vi "Main.vi"(8 "error in":errorcluster, 9 "Error Queue":refnum<queue>, 10 "Controller Queue":refnum<queue>, 11 "Application Events":refnum<user-event>) -> (0 "error out":errorcluster)   [LabVIEW 2020, in "User Console.lvlib"]
uses:
  User Console.lvlib
  Controller/Controls/Module Message.ctl
  Controller/Controls/Application Modules.ctl
  Controller/Controls/Application Event Message.ctl
  Controller/Controls/Application Events.ctl
  Controls/Module Loop Data.ctl
  Controller/Controller.lvlib
panel:
  in  "Door Buttons":cluster{"Door Open":bool, "Door Close":bool}
  in  "Floor Selection":T1
  in  "Elevator Call":T2
  in  "Emergency":bool
  # "[Covers: UI1]"
  # "[Covers: UI2]\n[Covers: UI2A] \n[Covers: UI2A1] \n[Covers: UI2A2] \n[Covers: UI2B] \n[Covers: UI2B1] \n[Covers: UI2B2] \n[Covers: UI2C] \n[Covers: UI2C1] \n[Covers: UI2C2] \n[Covers: UI2C3]"
  # "[Covers: UI2D] \n[Covers: UI2D1]"
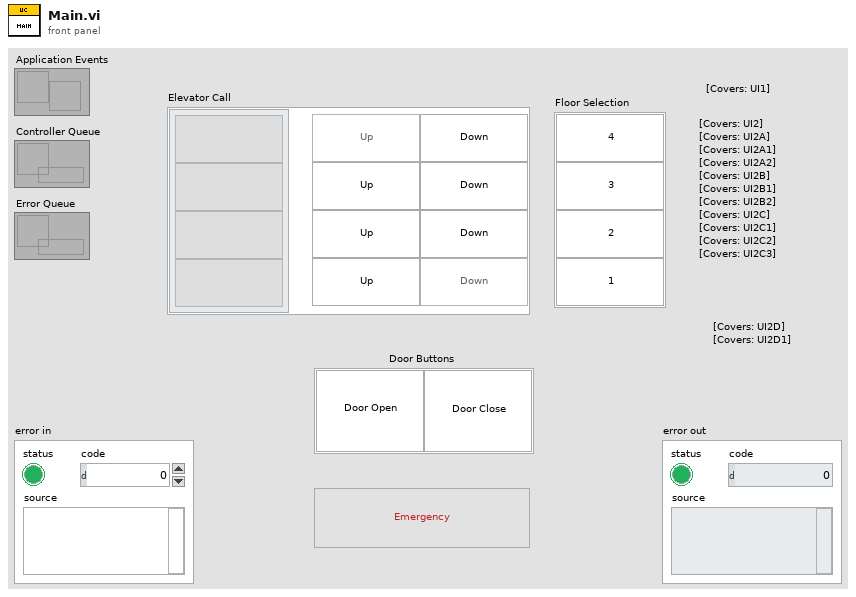
[diagram p1: front panel]
types:
  T1 = cluster{"Floor 1":bool, "Floor 2":bool, "Floor 3":bool, "Floor 4":bool}
  T2 = cluster{"Up Floor 1 ":bool, "Up Floor 2":bool, "Up Floor 3":bool, "Up Floor 4":bool, "Down Floor 1":bool, "Down Floor 2":bool, "Down Floor 3":bool, "Down Floor 4":bool, "Floors":string[]}
  T3 = typedef "Controller.lvlib/Application Events.ctl" = enum16{"Controller: Initialize", "Controller: Initialize Start And Move State", "Controller: Initialize Analysis State", "Controller: Initialize Continue Travel State", "Controller: Initialize Stop At Floor", "Controller: Initialize Open And Close Door Sequence", "Controller: Initialize No Request Remaining", "Controller: Initialize Emergency Call", "Controller: Initialize Terminate Process", "Controller: Publish State", "UI: Elevator Call", "UI: Broadcast State", "UI: Next Destination Reached", "UI: Timeout Reached", "UI: Emergency Call", "UI: Terminate State", "UI: Door Opened", "UI: Door Closed", "UI: Floor Reached", "UI: Door About To Close"}
  T4 = typedef "User Console.lvlib/Module Loop Data.ctl" = cluster{"Timing":cluster{"IsTiming?":bool, "Time Target Sec":dbl, "Time Ticks Ms":i32, "Time Ticks Counter":i32}}
  T5 = typedef "Controller.lvlib/Application Event Message.ctl" = cluster{"Source":T6, "Event":T3, "Data":variant}
  T6 = typedef "Controller.lvlib/Application Modules.ctl" = enum16{"Controller", "User Console", "Display Console", "Sensor Interface", "Configuration Database", "Error Module"}
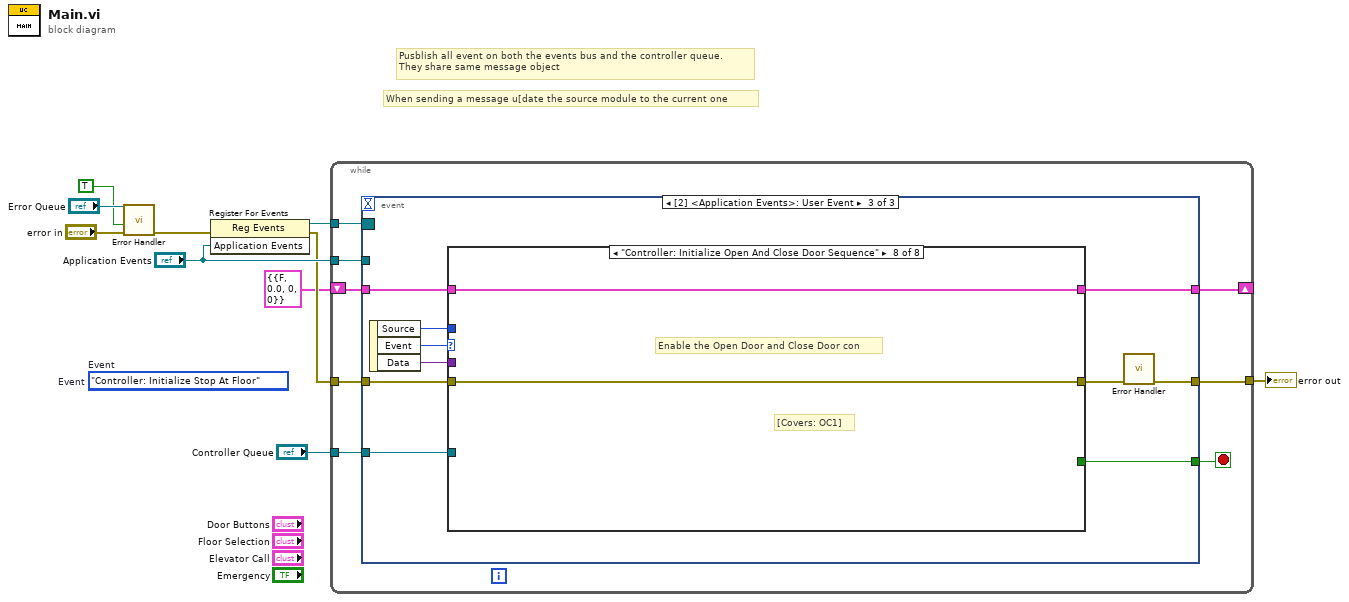
[diagram p0: block diagram]
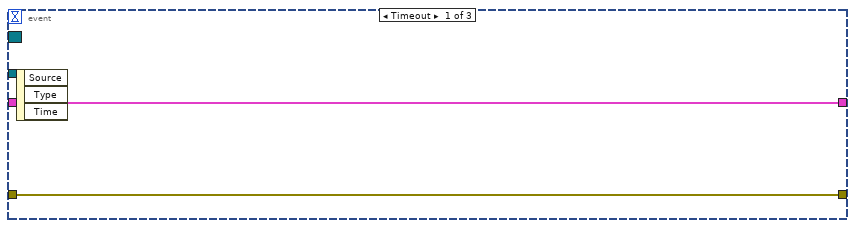
[diagram p2: hidden frame]
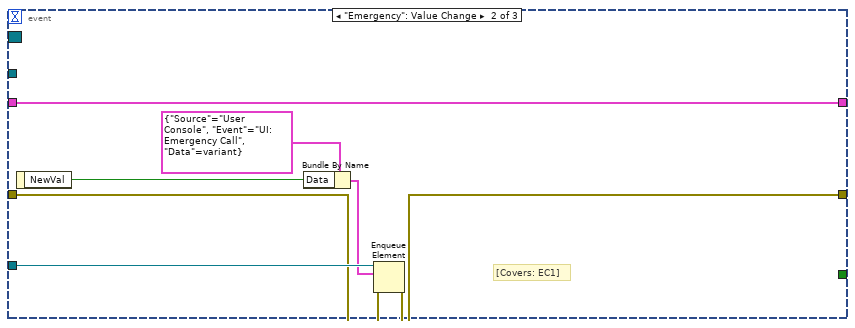
[diagram p3: hidden frame]
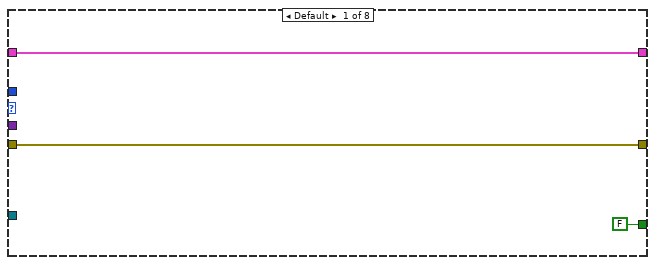
[diagram p4: hidden frame]
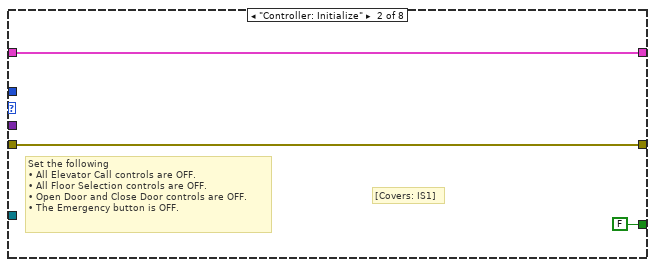
[diagram p5: hidden frame]
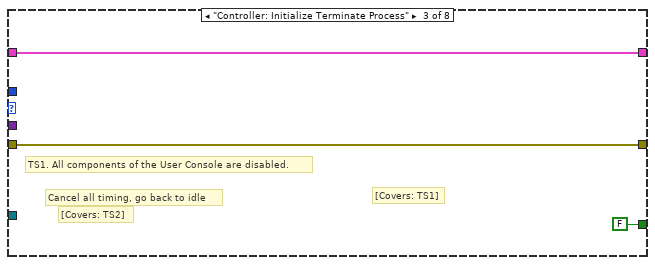
[diagram p6: hidden frame]
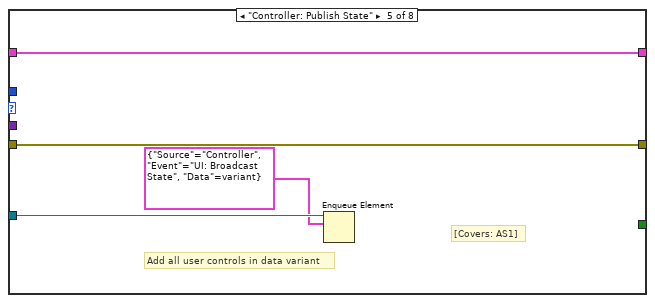
[diagram p8: hidden frame]
diagram:
  (unwired) Application_Events."Controller: Initialize Stop At Floor"  # Event
  (unwired) Application_Events."Controller: Initialize Stop At Floor"  # Event
  # "Pusblish all event on both the events bus and the controller queue. \nThey share same message object"
  # "When sending a message u[date the source module to the current one"
  n1 = call "Error Handler.vi"("error in"="error in", "Load Reference?"=TRUE, "Error Queue"="Error Queue") -> ("error out"=w4:errorcluster)  [unwired: 8 in]
  n2 = register-events(error in=w4, "Application Events") -> (reference out=w9:refnum<event-registration>, error out=w3:errorcluster)  [unwired: 1 in]
  n3 = while {
    tunnel: "Application Events" -> [w18]
    tunnel: w9 -> [w17]
    tunnel: w3 -> [w16]
    tunnel: "Controller Queue" -> [w15]
    tunnel: [w13] -> w2
    shift-right: [w11] -> _
    shift-left: T4 {"Timing"={"IsTiming?"=FALSE, "Time Target Sec"=0.0, "Time Ticks Ms"=0, "Time Ticks Counter"=0}} -> [w12]
    stop <- w14 stop-if-true
    n4 = event shown="[2] <Application Events>: User Event" {
      selector: w17 -> [_ _ _]
      dyn-events: _ -> [_ _ _]
      timeout: _ -> [_ _ _]
      tunnel: w18 -> [_ _ _]
      tunnel: w16 -> [w20 w26 w33]
      tunnel: w15 -> [_ w27 w28]
      tunnel: [_ _ w34] -> w14
      tunnel: [w20 w25 w31] -> w13
      tunnel: w12 -> [w19 w21 w30]
      tunnel: [w19 w21 w29] -> w11
      event Timeout {
        n5 = event-data() -> ()  [unwired: 1 in, 3 out]
      }
      event "Emergency": Value Change {
        # "[Covers: EC1]"
        n6 = event-data() -> ("NewVal"=w24:bool)  [unwired: 1 in]
        n7 = Bundle By Name(cluster=T5 {"Source"=enum."User Console", "Event"=enum."UI: Emergency Call", "Data"=variant} ("element"), "Data"=w24) -> (w22:T5)
        n8 = Enqueue Element(queue=w27, element=w22, error in (no error)=w26) -> (error out=w25:errorcluster)  [unwired: 1 in, 2 out]
      }
      event User Event {
        n9 = event-data() -> ("Source"=w36:T6, "Event"=w37:T3, "Data"=w35:variant)  [unwired: 1 in]
        n10 = case shown="\"Controller: Initialize Open And Close Door Sequence\"" w37 {
          tunnel: w36 -> [_ _ _ _ _ _ _ _]
          tunnel: w35 -> [_ _ _ _ _ _ _ _]
          tunnel: [FALSE FALSE FALSE _ _ _ _ _] -> w34
          tunnel: [w39 w42 w45 w48 w52 w54 w56 w58] -> w32
          tunnel: w33 -> [w39 w42 w45 w48 w52 w54 w56 w58]
          tunnel: w30 -> [w38 w41 w44 w47 w51 w53 w55 w57]
          tunnel: [w38 w41 w44 w47 w51 w53 w55 w57] -> w29
          tunnel: w28 -> [_ _ _ _ w50 _ _ _]
          frame Default {
          }
          frame "Controller: Initialize" {
            # "[Covers: IS1]"
            # "Set the following\n• All Elevator Call controls are OFF.\n• All Floor Selection controls are OFF.\n• Open Door and Close Door controls are OFF.\n• The Emergency button is OFF."
          }
          frame "Controller: Initialize Terminate Process" {
            # "Cancel all timing, go back to idle"
            # "[Covers: TS2]"
            # "[Covers: TS1]"
            # "TS1. All components of the User Console are disabled."
          }
          frame "Controller: Initialize No Request Remaining" {
          }
          frame "Controller: Publish State" {
            # "[Covers: AS1]"
            # "Add all user controls in data variant"
            n11 = Enqueue Element(queue=w50, element=T5 {"Source"=enum."Controller", "Event"=enum."UI: Broadcast State", "Data"=variant}) -> ()  [unwired: 2 in, 3 out]
          }
          frame "Controller: Initialize Stop At Floor" {
            # "[Covers: RF1] \n[Covers: RF2]"
            # "extract current floor from data variant"
            # "RF2. Turn the Elevator Call control OFF for the current floor and direction."
            # "RF1. Turn the Floor Selection control OFF for the current floor."
          }
          frame "Controller: Initialize Start And Move State" {
            # "Disable the Open Door and Close Door con"
            # "[Covers: SS1]"
          }
          frame "Controller: Initialize Open And Close Door Sequence" {
            # "[Covers: OC1]"
            # "Enable the Open Door and Close Door con"
          }
        }
        n12 = call "Error Handler.vi"("error in"=w32) -> ("error out"=w31:errorcluster)  [unwired: 10 in]
      }
    }
  }
  "error out" <- w2
